vi "Positions Cannot Contain a Beacon.vi"(0 "Beacons":set{T1}(c389), 1 "Y Row to Check":i32=10, 3 "Sensors":map{T1, T3}(c390), 4 "Boundary":T2) -> (5 "Positions Cannot Contain a Beacon":set{T1}(c389))   [LabVIEW 2020, in "AoC 2022.lvlib"]
uses:
  AoC 2022.lvlib
  Location.ctl
  Sensor Info.ctl
  Coverage Area.ctl
  <vilib>/Analysis/geometry.llb/Point in Polygon Position.ctl
  <vilib>/Analysis/geometry.llb/Point in Polygon (Scalar).vi
  <vilib>/Analysis/NI_AAL_Geometry.lvlib
  ce7427dc-c59f-493b-9153-69ee1a3bf334.vi
panel:
  out "size(s)":i32
  out "Positions Cannot Contain a Beacon":T1[](array[typedef])
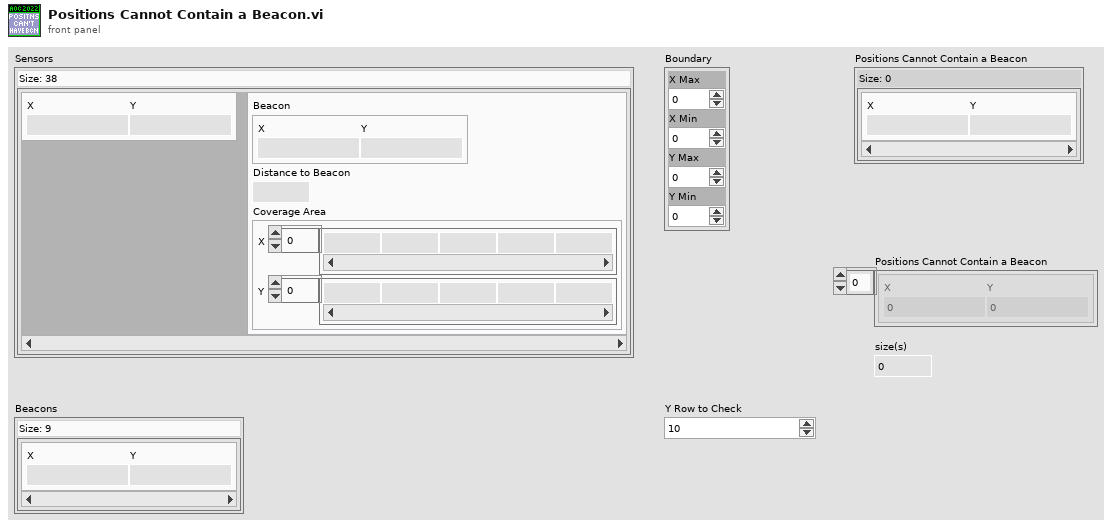
[diagram p1: front panel]
types:
  T1 = typedef "AoC 2022.lvlib/Location.ctl" = cluster{"X":i32, "Y":i32}
  T2 = cluster{"X Max":i32, "X Min":i32, "Y Max":i32, "Y Min":i32}
  T3 = typedef "AoC 2022.lvlib/Sensor Info.ctl" = cluster{"Beacon":T1, "Distance to Beacon":dbl, "Coverage Area":T4}
  T4 = typedef "AoC 2022.lvlib/Coverage Area.ctl" = cluster{"X":dbl[], "Y":dbl[]}
  T5 = typedef "NI_AAL_Geometry.lvlib/Point in Polygon Position.ctl" = u16
  T6 = cluster{"Points":cluster{"X":dbl, "Y":dbl}[], "Hole":bool}[]
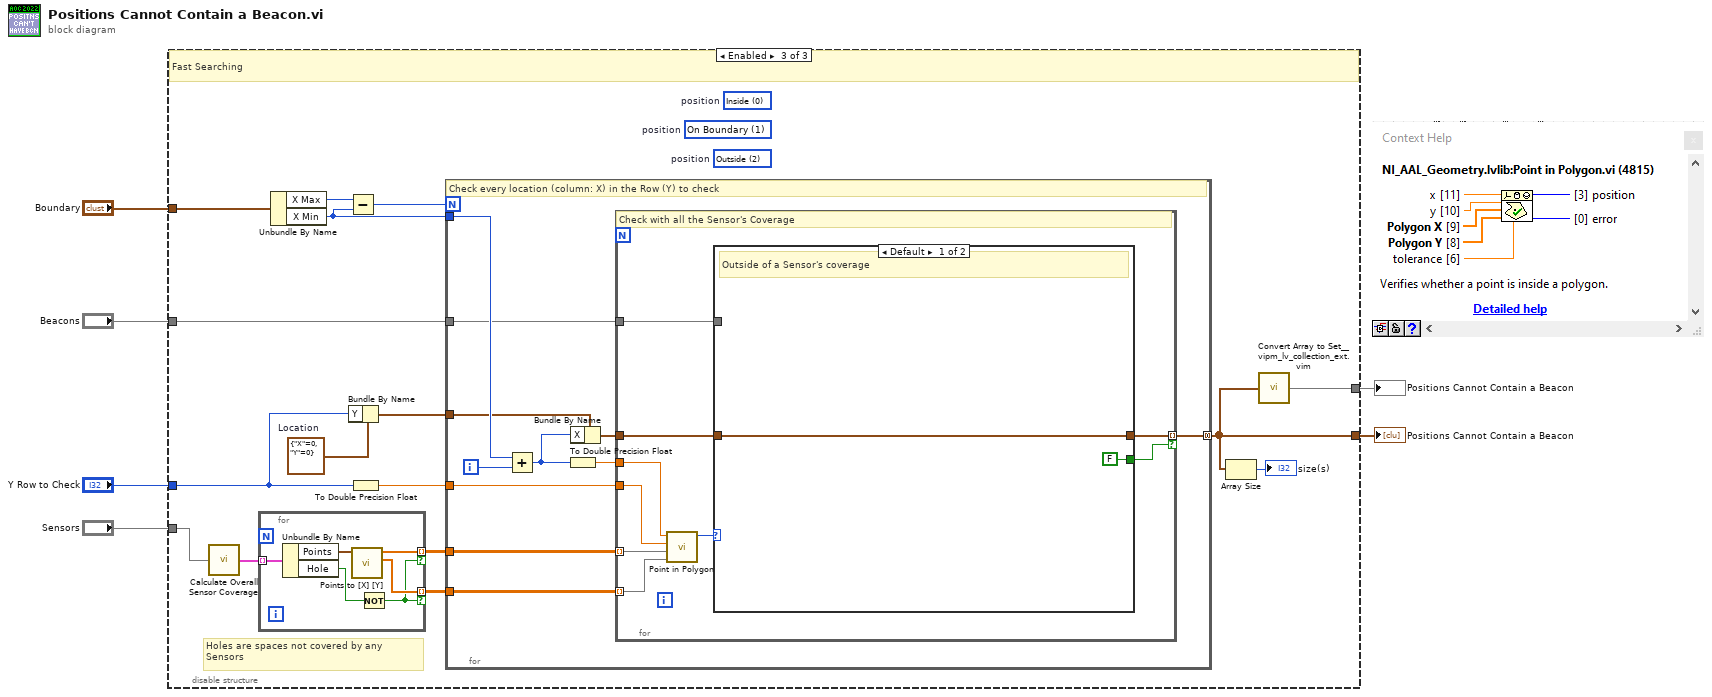
[diagram p0: block diagram]
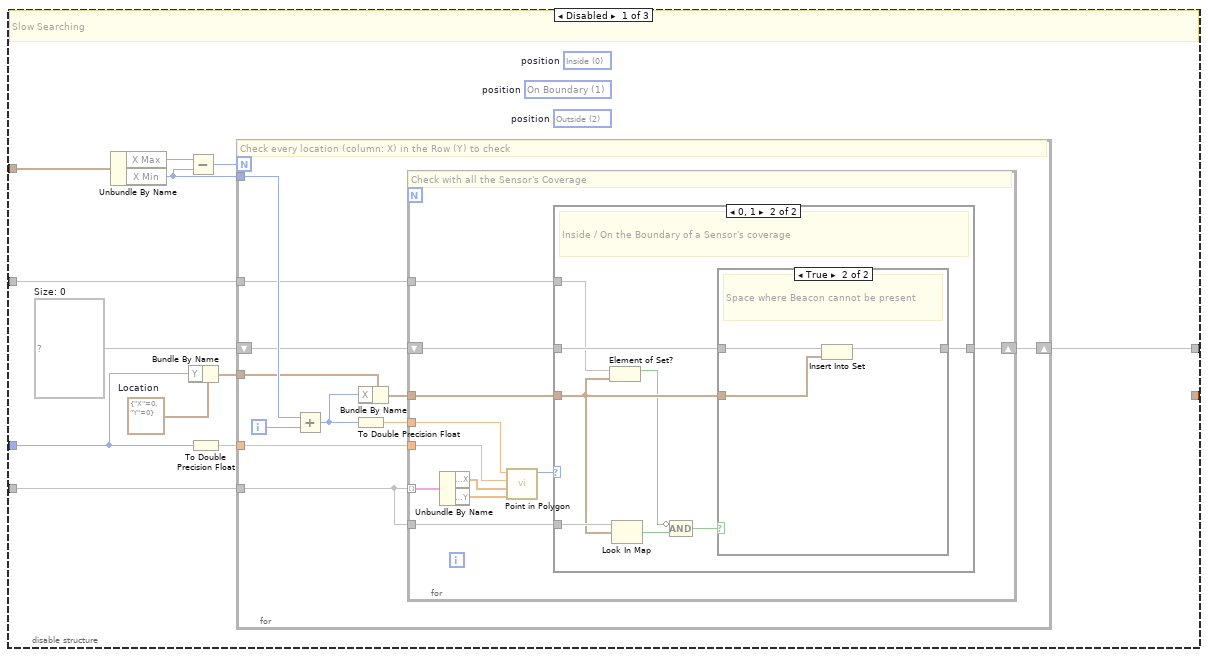
[diagram p2: hidden frame]
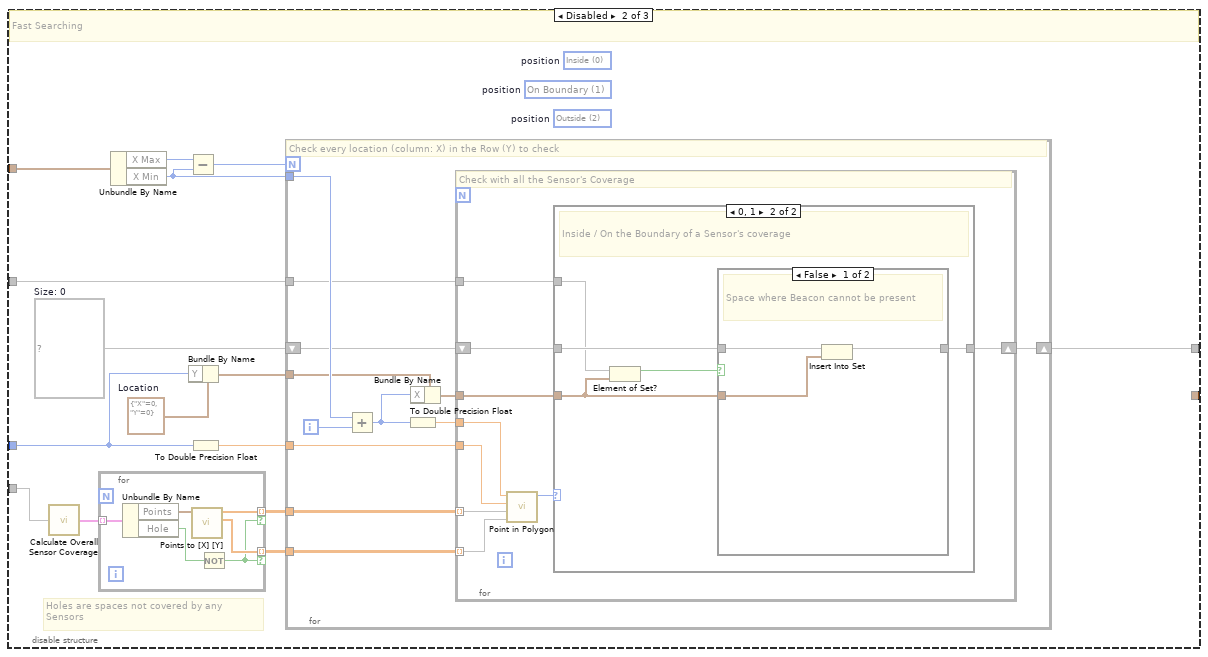
[diagram p5: hidden frame]
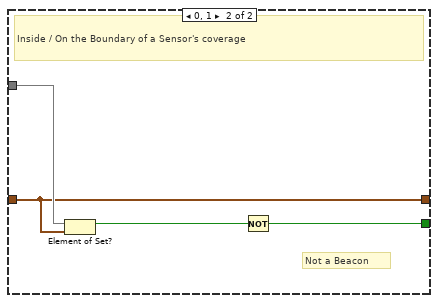
[diagram p8: hidden frame]
diagram:
  n1 = disable-structure shown="Enabled" {
    disable-tunnel: "Beacons" -> [w18 w68 w121]
    disable-tunnel: [w17 w67 w106] -> w5
    disable-tunnel: "Y Row to Check" -> [w15 w65 w119]
    disable-tunnel: "Boundary" -> [w9 w59 w114]
    disable-tunnel: "Sensors" -> [w7 w57 w112]
    disable-tunnel: [_ _ w107] -> w1
    frame Disabled {
      w14 = T1 {"X"=0, "Y"=0}  # Location
      w13 = set{T1} {}  # Size: 0
      (unwired) T5 0 items=["Inside", "On Boundary", "Outside"]  # position
      (unwired) T5 1 items=["Inside", "On Boundary", "Outside"]  # position
      (unwired) T5 2 items=["Inside", "On Boundary", "Outside"]  # position
      # "Slow Searching"
      n2 = Unbundle By Name(w9) -> ("X Max"=w10:i32, "X Min"=w12:i32)
      n3 = Subtract(x=w10, y=w12) -> (x-y=w11:i32)
      n4 = Bundle By Name(cluster=w14, "Y"=w15) -> (w16:T1)
      n5 = To Double Precision Float(number=w15) -> (double precision float=w8:dbl)
      n6 = for {
        N: w11 -> [_]
        tunnel: w12 -> [w29]
        tunnel: w7 -> [w19]
        tunnel: w8 -> [w27]
        shift-right: [w24] -> w17
        shift-left: w13 -> [w25]
        tunnel: w16 -> [w23]
        tunnel: w18 -> [w20]
        i -> [w26]
        # "Check every location (column: X) in the Row (Y) to check"
        n7 = Add(x=w29, y=w26) -> (x+y=w22:i32)
        n8 = To Double Precision Float(number=w22) -> (double precision float=w28:dbl)
        n9 = Bundle By Name(cluster=w23, "X"=w22) -> (w21:T1)
        n10 = for {
          tunnel: w19 -> [w40] mode=indexing
          tunnel: w28 -> [w37]
          tunnel: w27 -> [w36]
          shift-right: [w33] -> w24
          shift-left: w25 -> [w34]
          tunnel: w21 -> [w32]
          tunnel: w20 -> [w31]
          tunnel: w19 -> [w30]
          # "Check with all the Sensor's Coverage"
          n11 = Unbundle By Name(w40) -> ("Sensor Info.Coverage Area.X"=w38:dbl[], "Sensor Info.Coverage Area.Y"=w39:dbl[])
          n12 = call-poly <vilib>:"Point in Polygon.vi"("Polygon Y"=w39, "Polygon X"=w38, "y"=w36, "x"=w37) -> ("position"=w35:T5)  [unwired: 6 in, 1 out]
          n13 = case shown="0, 1" w35 {
            tunnel: w34 -> [w41 w49]
            tunnel: [w41 w48] -> w33
            tunnel: w32 -> [_ w45]
            tunnel: w31 -> [_ w46]
            tunnel: w30 -> [_ w47]
            frame Default {
              # "Outside of a Sensor's coverage"
            }
            frame 0, 1 {
              # "Inside / On the Boundary of a Sensor's coverage"
              n14 = Element of Set?(10:w45, 11:w46) -> (3:w43:bool)
              n15 = Look In Map(map=w47, key=w45) -> (key not found?=w44:bool)  [unwired: 1 in, 1 out]
              n16 = Compound Arithmetic op=AND(invert w43, w44) -> (w42:bool)
              n17 = case shown="True" w42 {
                tunnel: w49 -> [w50 w53]
                tunnel: [w50 w52] -> w48
                tunnel: w45 -> [_ w51]
                frame False {
                  # "It's another Sensor/Beacon"
                }
                frame True {
                  # "Space where Beacon cannot be present"
                  n18 = Insert Into Set(10:w51, 11:w53) -> (3:w52:set{T1})  [unwired: 1 out]
                }
              }
            }
          }
        }
      }
    }
    frame Disabled {
      w64 = T1 {"X"=0, "Y"=0}  # Location
      w63 = set{T1} {}  # Size: 0
      (unwired) T5 0 items=["Inside", "On Boundary", "Outside"]  # position
      (unwired) T5 1 items=["Inside", "On Boundary", "Outside"]  # position
      (unwired) T5 2 items=["Inside", "On Boundary", "Outside"]  # position
      # "Holes are spaces not covered by any Sensors"
      # "Fast Searching"
      n19 = call "Calculate Overall Sensor Coverage.vi"("Sensors"=w57) -> ("Overall Sensor Coverage"=w56:T6)
      n20 = for {
        tunnel: w56 -> [w74] mode=indexing
        tunnel: [w72] -> w55 mode=indexing if=w69
        tunnel: [w71] -> w54 mode=indexing if=w69
        n21 = Unbundle By Name(w74) -> ("Points"=w73:cluster{"X":dbl, "Y":dbl}[], "Hole"=w70:bool)
        n22 = call "Points to [X] [Y].vi"("Points"=w73) -> ("Y"=w71:dbl[], "X"=w72:dbl[])  [unwired: 9 in]
        n23 = Not(x=w70) -> (.not. x?=w69:bool)
      }
      n24 = Unbundle By Name(w59) -> ("X Max"=w60:i32, "X Min"=w62:i32)
      n25 = Subtract(x=w60, y=w62) -> (x-y=w61:i32)
      n26 = Bundle By Name(cluster=w64, "Y"=w65) -> (w66:T1)
      n27 = To Double Precision Float(number=w65) -> (double precision float=w58:dbl)
      n28 = for {
        N: w61 -> [_]
        tunnel: w62 -> [w86]
        tunnel: w58 -> [w84]
        shift-right: [w81] -> w67
        shift-left: w63 -> [w82]
        tunnel: w66 -> [w80]
        tunnel: w68 -> [w77]
        tunnel: w55 -> [w76]
        tunnel: w54 -> [w75]
        i -> [w83]
        # "Check every location (column: X) in the Row (Y) to check"
        n29 = Add(x=w86, y=w83) -> (x+y=w79:i32)
        n30 = To Double Precision Float(number=w79) -> (double precision float=w85:dbl)
        n31 = Bundle By Name(cluster=w80, "X"=w79) -> (w78:T1)
        n32 = for {
          tunnel: w85 -> [w95]
          tunnel: w84 -> [w94]
          shift-right: [w91] -> w81
          shift-left: w82 -> [w92]
          tunnel: w78 -> [w90]
          tunnel: w77 -> [w89]
          tunnel: w76 -> [w88] mode=indexing
          tunnel: w75 -> [w87] mode=indexing
          # "Check with all the Sensor's Coverage"
          n33 = call-poly <vilib>:"Point in Polygon.vi"("Polygon Y"=w87, "Polygon X"=w88, "y"=w94, "x"=w95) -> ("position"=w93:T5)  [unwired: 6 in, 1 out]
          n34 = case shown="0, 1" w93 {
            tunnel: w92 -> [w96 w101]
            tunnel: [w96 w100] -> w91
            tunnel: w90 -> [_ w98]
            tunnel: w89 -> [_ w99]
            frame Default {
              # "Outside of a Sensor's coverage"
            }
            frame 0, 1 {
              # "Inside / On the Boundary of a Sensor's coverage"
              n35 = Element of Set?(10:w98, 11:w99) -> (3:w97:bool)
              n36 = case shown="False" w97 {
                tunnel: w101 -> [w104 w105]
                tunnel: [w103 w105] -> w100
                tunnel: w98 -> [w102 _]
                frame False {
                  # "Space where Beacon cannot be present"
                  n37 = Insert Into Set(10:w102, 11:w104) -> (3:w103:set{T1})  [unwired: 1 out]
                }
                frame True {
                  # "It's another Beacon"
                }
              }
            }
          }
        }
      }
    }
    frame Enabled {
      w118 = T1 {"X"=0, "Y"=0}  # Location
      (unwired) T5 0 items=["Inside", "On Boundary", "Outside"]  # position
      (unwired) T5 1 items=["Inside", "On Boundary", "Outside"]  # position
      (unwired) T5 2 items=["Inside", "On Boundary", "Outside"]  # position
      # "Holes are spaces not covered by any Sensors"
      # "Fast Searching"
      n38 = call "Calculate Overall Sensor Coverage.vi"("Sensors"=w112) -> ("Overall Sensor Coverage"=w111:T6)
      n39 = for {
        tunnel: w111 -> [w127] mode=indexing
        tunnel: [w125] -> w110 mode=indexing if=w122
        tunnel: [w124] -> w109 mode=indexing if=w122
        n40 = Unbundle By Name(w127) -> ("Points"=w126:cluster{"X":dbl, "Y":dbl}[], "Hole"=w123:bool)
        n41 = call "Points to [X] [Y].vi"("Points"=w126) -> ("Y"=w124:dbl[], "X"=w125:dbl[])  [unwired: 9 in]
        n42 = Not(x=w123) -> (.not. x?=w122:bool)
      }
      n43 = Unbundle By Name(w114) -> ("X Max"=w115:i32, "X Min"=w117:i32)
      n44 = Subtract(x=w115, y=w117) -> (x-y=w116:i32)
      n45 = Bundle By Name(cluster=w118, "Y"=w119) -> (w120:T1)
      n46 = To Double Precision Float(number=w119) -> (double precision float=w113:dbl)
      n47 = for {
        N: w116 -> [_]
        tunnel: w117 -> [w138]
        tunnel: w113 -> [w136]
        tunnel: w120 -> [w134]
        tunnel: w121 -> [w131]
        tunnel: w110 -> [w130]
        tunnel: w109 -> [w129]
        tunnel: [w128] -> w107 mode=concatenating
        i -> [w135]
        # "Check every location (column: X) in the Row (Y) to check"
        n48 = Add(x=w138, y=w135) -> (x+y=w133:i32)
        n49 = To Double Precision Float(number=w133) -> (double precision float=w137:dbl)
        n50 = Bundle By Name(cluster=w134, "X"=w133) -> (w132:T1)
        n51 = for {
          tunnel: w137 -> [w147]
          tunnel: w136 -> [w146]
          tunnel: w132 -> [w144]
          tunnel: w131 -> [w143]
          tunnel: w130 -> [w142] mode=indexing
          tunnel: w129 -> [w141] mode=indexing
          tunnel: [w140] -> w128 mode=indexing if=w139
          # "Check with all the Sensor's Coverage"
          n52 = call-poly <vilib>:"Point in Polygon.vi"("Polygon Y"=w141, "Polygon X"=w142, "y"=w146, "x"=w147) -> ("position"=w145:T5)  [unwired: 6 in, 1 out]
          n53 = case shown="Default" w145 {
            tunnel: w144 -> [w149 w152]
            tunnel: w143 -> [_ w153]
            tunnel: [w149 w152] -> w140
            tunnel: [FALSE w150] -> w139
            frame Default {
              # "Outside of a Sensor's coverage"
            }
            frame 0, 1 {
              # "Not a Beacon"
              # "Inside / On the Boundary of a Sensor's coverage"
              n54 = Element of Set?(10:w152, 11:w153) -> (3:w151:bool)
              n55 = Not(x=w151) -> (.not. x?=w150:bool)
            }
          }
        }
      }
      n56 = Array Size(array=w107) -> (size(s)=→"size(s)":i32)
      n57 = call "Convert Array to Set__vipm_lv_collection_ext.vim"("array"=w107) -> ("set"=w106:set{T1})  [unwired: 6 in]
    }
  }
  "Positions Cannot Contain a Beacon" <- w5
  "Positions Cannot Contain a Beacon" <- w1
